vi "Close.vi"(8 "error in":errorcluster, 11 "AI DAQmx Cont CFG in":refnum<class "AI DAQmx Cont CFG.lvclass">) -> (0 "error out":errorcluster, 3 "AI DAQmx Cont CFG out":refnum<class "AI DAQmx Cont CFG.lvclass">)   [LabVIEW 2023, in "AI DAQmx Cont CFG.lvclass"]
uses:
  AI DAQmx Cont CFG.lvclass
  AI DAQmx Cont CFG.lvclass/AI DAQmx Cont CFG.ctl
  DAQmx/DAQmx Base CFG/DAQmx Base CFG.lvclass
  DAQmx/BufferLastReadingsDBL/BufferLastReadings DBL.lvclass
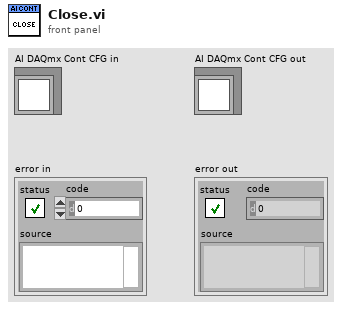
[diagram p1: front panel]
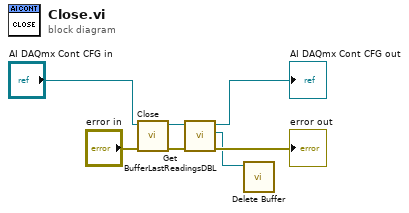
[diagram p0: block diagram]
diagram:
  n1 = call-parent "Close.vi"("error in"="error in", "DAQmx Base CFG in"="AI DAQmx Cont CFG in") -> ("error out"=→"error out":errorcluster, "DAQmx Base CFG out"=w3:refnum<class "AI DAQmx Cont CFG.lvclass">)  [unwired: 8 in]
  n2 = call "Get BufferLastReadingsDBL.vi"("AI DAQmx Cont CFG in"=w3) -> ("BufferLastReadings DBL"=w2:refnum<class "BufferLastReadings DBL.lvclass">, "AI DAQmx Cont CFG out"=→"AI DAQmx Cont CFG out":refnum<class "AI DAQmx Cont CFG.lvclass">)  [unwired: 9 in]
  n3 = call "Delete Buffer.vi"("BufferLastReadings DBL in"=w2) -> ()  [unwired: 10 in, 1 out]
